vi "H.vi"(9 "Z":u32 format="%08x", 10 "Y":u32 format="%08x", 11 "X":u32 format="%08x") -> (3 "H":u32 format="%08x")   [LabVIEW 2013, in "MD5.lvlib" / "MD5.lvclass"]
uses:
  MD5.lvclass
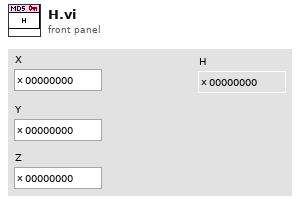
[diagram p1: front panel]
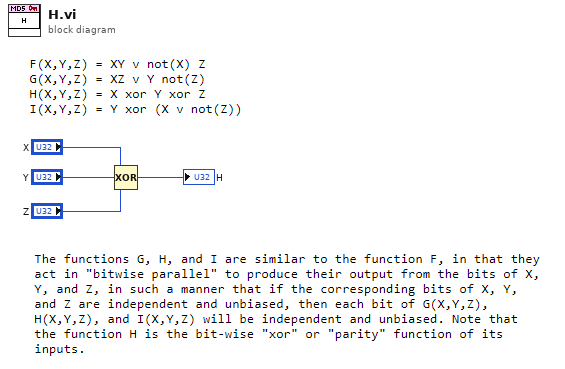
[diagram p0: block diagram]
diagram:
  n1 = Compound Arithmetic op=XOR("X", "Y", "Z") -> (→"H":u32)
